vi "Create Pattern Script - Rd Compare Frame.vi"(8 "error in (no error)":errorcluster, 10 "FRM Data":T1 {"Addr" format="%x"; "Data" format="%x"}, 11 "SPI 3W Pattern Creator in":refnum<class "SPI 3W Pattern Creator.lvclass">) -> (0 "error out":errorcluster, 2 "String":string, 3 "SPI 3W Pattern Creator out":refnum<class "SPI 3W Pattern Creator.lvclass">)   [LabVIEW 2018, in "SPI 3W Pattern Creator.lvlib" / "SPI 3W Pattern Creator.lvclass"]
uses:
  SPI 3W Pattern Creator.lvclass
  Ctls/Frame Data - SPI_3W.ctl
  Ctls/RW Options.ctl
  Protocols/SPI Root Pattern Creator.lvlibp/Plugins/SouceCode/SPI_Pattern Creator/SPI Root/Data Type.ctl
  Protocols/SPI Root Pattern Creator.lvlibp/Plugins/SouceCode/SPI_Pattern Creator/SPI Root/Special Frame Type.ctl
  Protocols/SPI Root Pattern Creator.lvlibp/Plugins/SouceCode/SPI_Pattern Creator/SPI Root/SPI Root Pattern Creator.lvclass
  C:/P4 Workspace/PC Client/Solutions/5g_eap/trunk/1.0/HiSi5GmmWave/Pattern_Gen_Tool/Plugins/Protocols/SPI Root Pattern Creator.lvlibp/Plugins/SouceCode/SPI_Pattern Creator/SPI Root/SPI Root Pattern Creator.lvclass
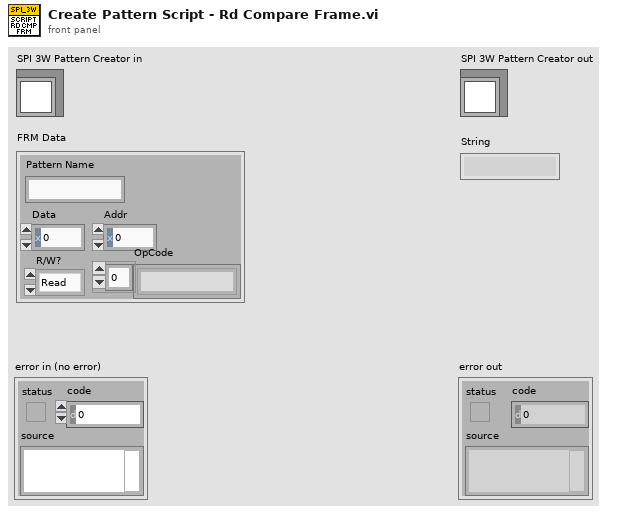
[diagram p1: front panel]
types:
  T1 = typedef "Frame Data - SPI_3W.ctl" = cluster{"Pattern Name":string, "Data":u16, "Addr":u16, "OpCode":string[], "R/W?":T2}
  T2 = typedef "RW Options.ctl" = enum16{"Read", "Write", "R/W"}
  T3 = typedef "SPI Root Pattern Creator.lvlibp/SPI Root Pattern Creator.lvclass/Special Frame Type.ctl" = enum16{"SPI 4W FRM Start", "SPI 4W Wait", "SPI 4W FRM End", "SPI 4W Write Cmd", "SPI Rd Collect Cmd", "SPI Rd Value Cmd", "SPI 3W FRM Start", "SPI 3W Write Cmd", "SPI 3W FRM End", "SPI 3W Wait", "SPI 3W Rd Cmd"}
  T4 = typedef "SPI Root Pattern Creator.lvlibp/SPI Root Pattern Creator.lvclass/Data Type.ctl" = enum16{"Drive", "Compare", "Read"}
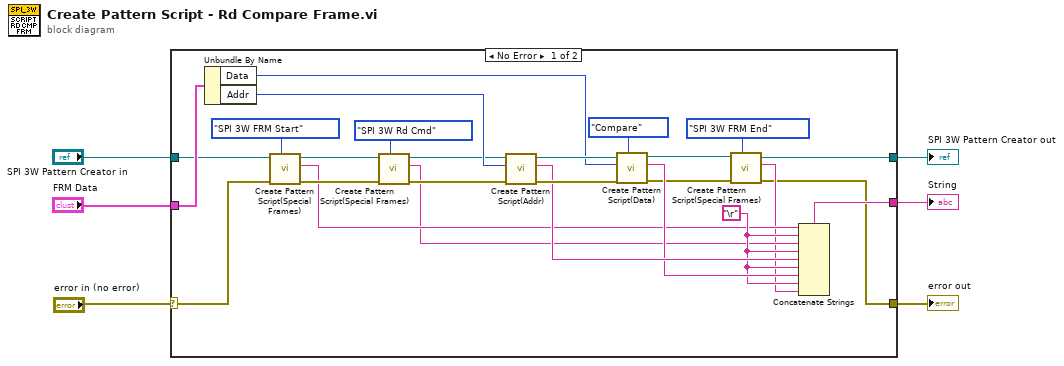
[diagram p0: block diagram]
diagram:
  n1 = case shown="No Error" "error in (no error)" {
    selector: "error in (no error)" -> [w23 w34]
    tunnel: "SPI 3W Pattern Creator in" -> [w22 w33]
    tunnel: "FRM Data" -> [w32 _]
    tunnel: [w12 w33] -> w3
    tunnel: [w10 w34] -> w2
    tunnel: [w24 _] -> w1
    frame No Error {
      w25 = "\r"
      n2 = Unbundle By Name(w32) -> ("Data"=w28:u16, "Addr"=w31:u16)
      n3 = call "Create Pattern Script(Special Frames).vi"("Special Frame Type"=Special_Frame_Type."SPI 3W FRM Start", "error in (no error)"=w23, "SPI Root Pattern Creator in"=w22) -> ("error out"=w19:errorcluster, "String out"=w18:string, "SPI Root Pattern Creator out"=w21:refnum<class "SPI 3W Pattern Creator.lvclass">)  [unwired: 6 in]
      n4 = call "Create Pattern Script(Special Frames).vi"("Special Frame Type"=Special_Frame_Type."SPI 3W Rd Cmd", "error in (no error)"=w19, "SPI Root Pattern Creator in"=w21) -> ("error out"=w17:errorcluster, "String out"=w16:string, "SPI Root Pattern Creator out"=w20:refnum<class "SPI 3W Pattern Creator.lvclass">)  [unwired: 6 in]
      n5 = call-dynamic "Create Pattern Script(Addr).vi"("error in (no error)"=w17, "Addr"=w31, "SPI 3W Pattern Creator in"=w20) -> ("error out"=w30:errorcluster, "String"=w27:string, "SPI 3W Pattern Creator out"=w29:refnum<class "SPI 3W Pattern Creator.lvclass">)  [unwired: 6 in]
      n6 = call-dynamic "Create Pattern Script(Data).vi"("Data Type"=Data_Type."Compare", "error in (no error)"=w30, "Data"=w28, "SPI 3W Pattern Creator in"=w29) -> ("error out"=w13:errorcluster, "String"=w26:string, "SPI 3W Pattern Creator out"=w14:refnum<class "SPI 3W Pattern Creator.lvclass">)  [unwired: 5 in]
      n7 = call "Create Pattern Script(Special Frames).vi"("Special Frame Type"=Special_Frame_Type."SPI 3W FRM End", "error in (no error)"=w13, "SPI Root Pattern Creator in"=w14) -> ("error out"=w10:errorcluster, "String out"=w11:string, "SPI Root Pattern Creator out"=w12:refnum<class "SPI 3W Pattern Creator.lvclass">)  [unwired: 6 in]
      n8 = Concatenate Strings(w18, w25, w16, w25, w27, w25, w26, w25, w11) -> (w24:string)
    }
    frame Error {
    }
  }
  "error out" <- w2
  "SPI 3W Pattern Creator out" <- w3
  "String" <- w1
